vi "Type to String.vi"(7 "application reference (local)":refnum<vi>, 8 "Error In":errorcluster, 11 "Type":variant) -> (0 "Error Out":errorcluster, 3 "String":string)   [LabVIEW 2015, in "Scripting.lvlib"]
uses:
  Scripting.lvlib
  <vilib>/Utility/Data Type/NI_Data Type.lvlib
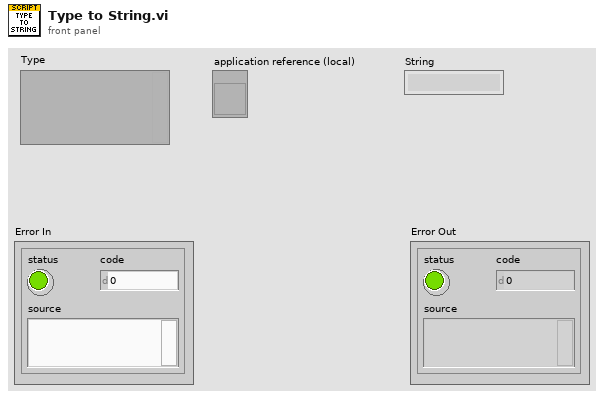
[diagram p1: front panel]
types:
  T1 = typedef "NI_Data Type.lvlib/Data Type.ctl" = enum8{"Invalid Type", "Void", "I8", "I16", "I32", "I64", "U8", "U16", "U32", "U64", "Single Float", "Double Float", "Extended Float", "Single Complex", "Double Complex", "Extended Complex", "Enum U8", "Enum U16", "Enum U32", "Enum U64", "Single Float With Unit", "Double Float With Unit", "Extended Float With Unit", "Single Complex with Unit", "Double Complex with Unit", "Extended Complex with Unit", "Boolean", "String", "Path", "Picture", "Tag", "Array", "Cluster", "Variant", "LV Variant", "Waveform", "Timestamp", "Digital Waveform", "Digital Data", "ExpressData", "Refnum", "External Data", "VI", "Poly VI", "LabVIEW Class Instance", "Fixed Point"}
  T2 = typedef "NI_Data Type.lvlib/Type Definition Info.ctl" = cluster{"Name":string, "Timestamp":u32}
  T3 = cluster{"Unit Type":enum8{"Radians", "Steradians", "Seconds", "Meters", "Kilograms", "Amperes", "Kelvins", "Moles", "Candelas", "InvalidUnit"}, "Exponent":i8}[]
  T4 = cluster{"Type":enum8{"Variable", "Fixed", "Bounded"}, "Size":u32}[]
  T5 = typedef "NI_Data Type.lvlib/Unit Info.ctl" = cluster{"Unit Type":T6, "Exponent":i16}
  T6 = typedef "NI_Data Type.lvlib/Unit Type.ctl" = enum16{"Radians", "Steradians", "Seconds", "Meters", "Kilograms", "Amperes", "Kelvins", "Moles", "Candelas", "InvalidUnit"}
  T7 = typedef "NI_Data Type.lvlib/Memory Info.ctl" = cluster{"Type":T8, "Size":u32}
  T8 = typedef "NI_Data Type.lvlib/Memory Type.ctl" = enum16{"Variable", "Fixed", "Bounded"}
  T9 = cluster{"string":string, string, "string":string}
  T10 = typedef "LVFixedPointRepRangeTypeDef.ctl" = cluster{"Range Min":dbl, "Range Max":dbl, "Delta":dbl}
  T11 = typedef "LVFixedPointRepBitsTypeDef.ctl" = cluster{"Signed":bool, "Word Length":u32, "Integer Word Length":i32}
  T12 = cluster{"FXP Representation":T11, "FXP Range":T10, "Include Overflow Status?":bool}
  T13 = typedef "NI_Data Type.lvlib/Tag Type.ctl" = enum16{"kNoTagType", "\tkDSCTagType", "\tkOldDAQTagType", "\tkIVITagType", "\tkVISATagType", "\tkGenClassTagType", "\tkUnusedTagType1", "\tkFPTagType", "\tkMotionTagType", "\tkDAQmxTaskTagType", "\tkDAQmxChannelTagType", "\tkDAQmxScaleTagType", "\tkDAQmxDeviceTagType", "\tkDAQmxTerminalTagType", "\tkDAQmxPhysChanTagType", "\tkDAQmxTriggerTagType", "\tkDAQmxSwitchTagType", "\tkDAQmxSignalTagType", "\tkUnusedTagType2", "\tkCANTaskTagType", "\tkCANInterfaceTagType", "\tkCANChannelTagType", "\tkNumTagTypes"}
  T14 = typedef "NI_Data Type.lvlib/Refnum Type.ctl" = enum16{"NotARefnum", "UnknownRefnum", "Generic", "Datalog", "ByteStream", "Device", "Occurence", "TCPNetConnection", "Auto", "Menu", "Imaq", "Hardware", "DataSocket", "Visa", "IVI", "UDPNetConnection", "Notifier", "Queue", "Irda", "EventReg", "DotNet", "UserEvent", "Callback", "UNUSED_EMPTY_POSITION", "BlueToothNetConnection", "LVObjApp", "LVObjVI", "LVObjUnknown", "GenericClass", "UserDefinedRefnumTag", "DataValue", "RT FIFO", "TDMS File"}
  T15 = typedef "NI_Data Type.lvlib/VI Info.ctl" = cluster{"Connector Pane Pattern":i16, "Connector Pane Rotation":i16, "Flags":u32[], "Modification Date":timestamp, "Asynchronous":bool, "Non-Function":bool, "Subroutine":bool, "SubSystem":bool}
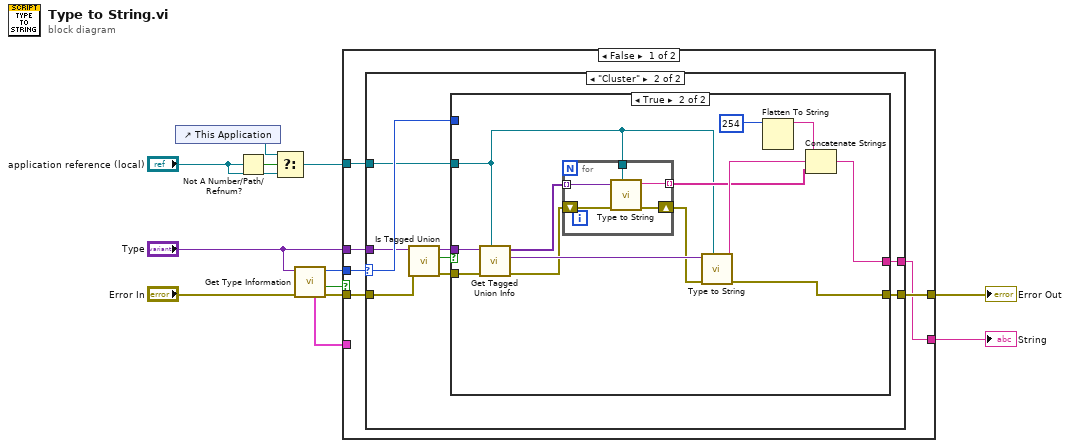
[diagram p0: block diagram]
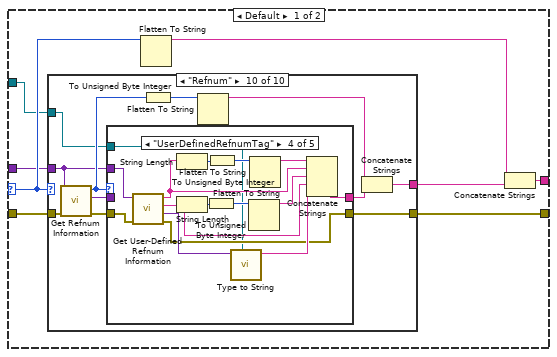
[diagram p2: hidden frame]
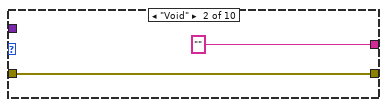
[diagram p4: hidden frame]
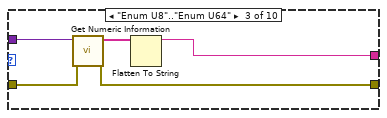
[diagram p5: hidden frame]
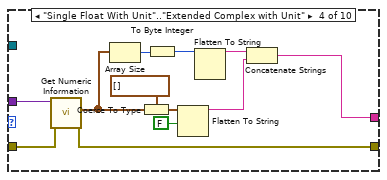
[diagram p6: hidden frame]
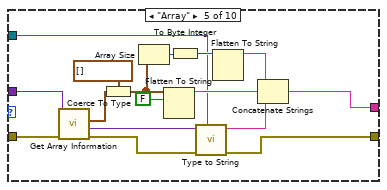
[diagram p7: hidden frame]
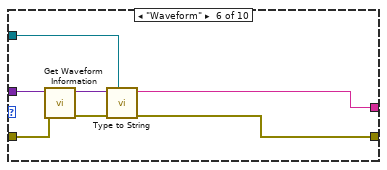
[diagram p8: hidden frame]
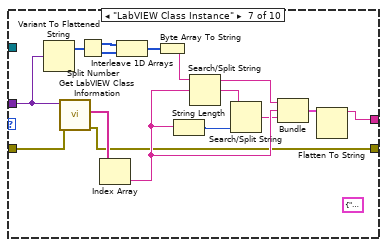
[diagram p9: hidden frame]
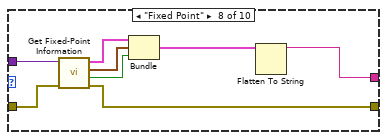
[diagram p10: hidden frame]
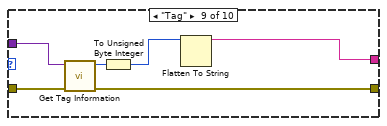
[diagram p11: hidden frame]
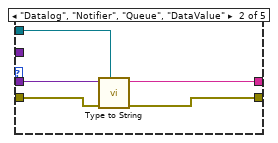
[diagram p13: hidden frame]
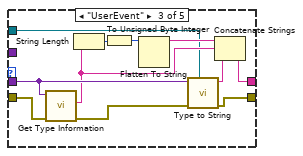
[diagram p14: hidden frame]
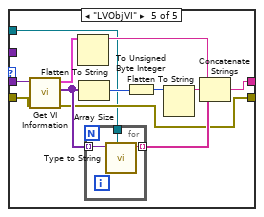
[diagram p15: hidden frame]
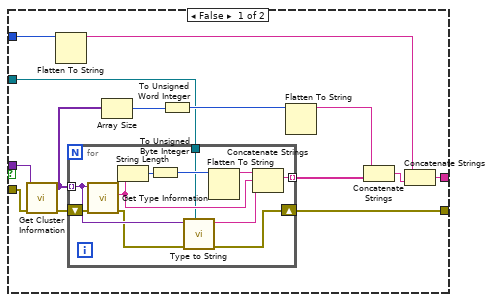
[diagram p16: hidden frame]
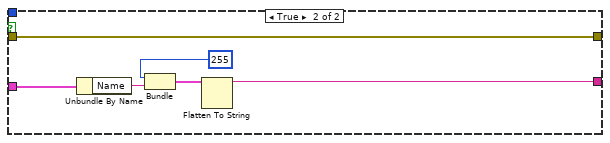
[diagram p17: hidden frame]
diagram:
  n1 = control-ref of="This Application"() -> (w3:refnum<vi>)
  n2 = Not A Number/Path/Refnum?(number/path/refnum="application reference (local)") -> (NaN/Path/Refnum?=w4:bool)
  n3 = Select(t=w3, s=w4, f="application reference (local)") -> (s? t:f=w1:refnum<vi>)
  n4 = call <vilib>:"Get Type Information.vi"("error in (no error)"="Error In", "Variant"="Type") -> ("error out"=w7:errorcluster, "Type Definition"=w11:bool, "Type"=w8:T1, "Type Definition Info"=w10:T2)  [unwired: 5 in, 1 out]
  n5 = case shown="False" w11 {
    tunnel: w10 -> [_ w215]
    tunnel: "Type" -> [w17 _]
    tunnel: w8 -> [w18 _]
    tunnel: w7 -> [w15 w210]
    tunnel: [w14 w211] -> w5
    tunnel: [w16 w210] -> w6
    tunnel: w1 -> [w13 _]
    frame False {
      n6 = case shown="\"Cluster\"" w18 {
        selector: w18 -> [w24 w164]
        tunnel: w17 -> [w20 w161]
        tunnel: [w26 w166] -> w16
        tunnel: w15 -> [w25 w165]
        tunnel: [w21 w163] -> w14
        tunnel: w13 -> [w19 w158]
        frame Default {
          n7 = case shown="\"Refnum\"" w24 {
            tunnel: [w27 w29 w30 w44 w58 w64 w70 w86 w98 w102] -> w26
            tunnel: w25 -> [w27 w29 w31 w45 w62 w69 w85 w92 w99 w110]
            tunnel: [_ "" w34 w35 w55 w65 w83 w87 w94 w104] -> w23
            tunnel: w20 -> [_ _ w33 w46 w61 w68 w82 w93 w97 w101]
            tunnel: w19 -> [_ _ _ _ w47 w63 _ _ _ w100]
            frame Default {
            }
            frame "Void" {
            }
            frame "Enum U8".."Enum U64" {
              n8 = call <vilib>:"Get Numeric Information.vi"("error in (no error)"=w31, "Variant"=w33) -> ("error out"=w30:errorcluster, "Enum Names"=w32:string[])  [unwired: 6 in, 2 out]
              n9 = Flatten To String(anything=w32) -> (data string=w34:string)  [unwired: 3 in, 2 out]
            }
            frame "Single Float With Unit".."Extended Complex with Unit" {
              n10 = call <vilib>:"Get Numeric Information.vi"("error in (no error)"=w45, "Variant"=w46) -> ("error out"=w44:errorcluster, "Units"=w40:T5[])  [unwired: 6 in, 2 out]
              n11 = Array Size(array=w40) -> (size(s)=w39:i32)
              n12 = Coerce To Type(0:w40, 1:T3 [] ("type")) -> (2:w42:T3)
              n13 = To Byte Integer(number=w39) -> (8bit integer=w38:i8)
              n14 = Flatten To String(anything=w42, prepend array or string size? (T)=FALSE) -> (data string=w36:string)  [unwired: 2 in, 2 out]
              n15 = Flatten To String(anything=w38) -> (data string=w37:string)  [unwired: 3 in, 2 out]
              n16 = Concatenate Strings(w37, w36) -> (w35:string)
            }
            frame "Array" {
              n17 = call <vilib>:"Get Array Information.vi"("error in (no error)"=w62, "Variant"=w61) -> ("error out"=w59:errorcluster, "Array Element Data Type"=w60:variant, "Array Lengths"=w54:T7[])  [unwired: 6 in, 1 out]
              n18 = Coerce To Type(0:w54, 1:T4 [] ("Array Lengths")) -> (2:w51:T4)
              n19 = Array Size(array=w51) -> (size(s)=w50:i32)
              n20 = Flatten To String(anything=w51, prepend array or string size? (T)=FALSE) -> (data string=w57:string)  [unwired: 2 in, 2 out]
              n21 = To Byte Integer(number=w50) -> (8bit integer=w49:i8)
              n22 = call "Type to String.vi"("application reference (local)"=w47, "Error In"=w59, "Type"=w60) -> ("Error Out"=w58:errorcluster, "String"=w56:string)  [unwired: 7 in]
              n23 = Flatten To String(anything=w49) -> (data string=w48:string)  [unwired: 3 in, 2 out]
              n24 = Concatenate Strings(w48, w57, w56) -> (w55:string)
            }
            frame "Waveform" {
              n25 = call <vilib>:"Get Waveform Information.vi"("error in (no error)"=w69, "Variant"=w68) -> ("error out"=w66:errorcluster, "Y Array Type"=w67:variant)  [unwired: 8 in]
              n26 = call "Type to String.vi"("application reference (local)"=w63, "Error In"=w66, "Type"=w67) -> ("Error Out"=w64:errorcluster, "String"=w65:string)  [unwired: 7 in]
            }
            frame "LabVIEW Class Instance" {
              (unwired) T9 {"string"="", "", "string"=""} ("output cluster")
              n27 = Variant To Flattened String(Variant=w82) -> (1:w81:i16[])  [unwired: 1 out]
              n28 = call <vilib>:"Get LabVIEW Class Information.vi"("error in (no error)"=w85, "Variant"=w82) -> ("error out"=w70:errorcluster, "Qualified LabVIEW Class Name"=w84:string[])  [unwired: 7 in, 1 out]
              n29 = Split Number(x=w81) -> (hi(x)=w80:u8[], lo(x)=w79:u8[])
              n30 = Index Array(array=w84) -> (element=w73:string)  [unwired: 1 in]
              n31 = Interleave 1D Arrays(w80, w79) -> (w78:u8[])
              n32 = Byte Array To String(unsigned byte array=w78) -> (string=w77:string)
              n33 = String Length(string=w73) -> (length=w75:i32)
              n34 = Search/Split String(string=w77, search string/char (-)=w73) -> (substring before match=w74:string, match + rest of string=w76:string)  [unwired: 1 in, 1 out]
              n35 = Search/Split String(string=w76, offset (0)=w75) -> (match + rest of string=w72:string)  [unwired: 1 in, 2 out]
              n36 = Bundle("string"=w74, w73, "string"=w72) -> (w71:T9)  [unwired: 1 in]
              n37 = Flatten To String(anything=w71) -> (data string=w83:string)  [unwired: 3 in, 2 out]
            }
            frame "Fixed Point" {
              n38 = call <vilib>:"Get Fixed-Point Information.vi"("error in (no error)"=w92, "Variant"=w93) -> ("error out"=w86:errorcluster, "Include Overflow Status?"=w89:bool, "FXP Range"=w90:T10, "FXP Representation"=w91:T11)  [unwired: 6 in]
              n39 = Bundle("FXP Representation"=w91, "FXP Range"=w90, "Include Overflow Status?"=w89) -> (w88:T12)  [unwired: 1 in]
              n40 = Flatten To String(anything=w88) -> (data string=w87:string)  [unwired: 3 in, 2 out]
            }
            frame "Tag" {
              n41 = call <vilib>:"Get Tag Information.vi"("error in (no error)"=w99, "Variant"=w97) -> ("error out"=w98:errorcluster, "Tag Type"=w96:T13)  [unwired: 8 in]
              n42 = To Unsigned Byte Integer(number=w96) -> (unsigned 8bit integer=w95:u8)
              n43 = Flatten To String(anything=w95) -> (data string=w94:string)  [unwired: 3 in, 2 out]
            }
            frame "Refnum" {
              n44 = call <vilib>:"Get Refnum Information.vi"("error in (no error)"=w110, "Variant"=w101) -> ("error out"=w107:errorcluster, "Strict Type"=w106:variant, "Reference Type"=w109:T14)  [unwired: 6 in, 1 out]
              n45 = case shown="\"UserDefinedRefnumTag\"" w109 {
                tunnel: w107 -> [w111 w115 w127 w142 w147]
                tunnel: w106 -> [_ w116 w124 _ w146]
                tunnel: [_ w114 w119 w131 w145] -> w103
                tunnel: [w111 w113 w126 w130 w144] -> w102
                tunnel: w101 -> [_ _ _ w129 _]
                tunnel: w100 -> [_ w112 w117 w128 w143]
                frame Default {
                }
                frame "Datalog", "Notifier", "Queue", "DataValue" {
                  n46 = call "Type to String.vi"("application reference (local)"=w112, "Error In"=w115, "Type"=w116) -> ("Error Out"=w113:errorcluster, "String"=w114:string)  [unwired: 7 in]
                }
                frame "UserEvent" {
                  n47 = call <vilib>:"Get Type Information.vi"("error in (no error)"=w127, "Variant"=w124) -> ("error out"=w125:errorcluster, "Name"=w121:string)  [unwired: 5 in, 3 out]
                  n48 = String Length(string=w121) -> (length=w123:i32)
                  n49 = To Unsigned Byte Integer(number=w123) -> (unsigned 8bit integer=w118:u8)
                  n50 = Flatten To String(anything=w118) -> (data string=w122:string)  [unwired: 3 in, 2 out]
                  n51 = call "Type to String.vi"("application reference (local)"=w117, "Error In"=w125, "Type"=w124) -> ("Error Out"=w126:errorcluster, "String"=w120:string)  [unwired: 7 in]
                  n52 = Concatenate Strings(w122, w121, w120) -> (w119:string)
                }
                frame "UserDefinedRefnumTag" {
                  n53 = call <vilib>:"Get User-Defined Refnum Information.vi"("error in (no error)"=w142, "Variant"=w129) -> ("error out"=w130:errorcluster, "User Data"=w141:variant, "Type Name"=w133:string, "Class Name"=w135:string)  [unwired: 6 in]
                  n54 = String Length(string=w135) -> (length=w138:i32)
                  n55 = String Length(string=w133) -> (length=w137:i32)
                  n56 = To Unsigned Byte Integer(number=w137) -> (unsigned 8bit integer=w139:u8)
                  n57 = To Unsigned Byte Integer(number=w138) -> (unsigned 8bit integer=w140:u8)
                  n58 = call "Type to String.vi"("application reference (local)"=w128, "Type"=w141) -> ("String"=w132:string)  [unwired: 8 in, 1 out]
                  n59 = Flatten To String(anything=w139) -> (data string=w134:string)  [unwired: 3 in, 2 out]
                  n60 = Flatten To String(anything=w140) -> (data string=w136:string)  [unwired: 3 in, 2 out]
                  n61 = Concatenate Strings(w136, w135, w134, w133, w132) -> (w131:string)
                }
                frame "LVObjVI" {
                  n62 = call <vilib>:"Get VI Information.vi"("error in (no error)"=w147, "Variant"=w146) -> ("error out"=w144:errorcluster, "VI Terminal Types"=w149:variant[], "VI Info"=w148:T15)  [unwired: 6 in, 1 out]
                  n63 = Flatten To String(anything=w148) -> (data string=w152:string)  [unwired: 3 in, 2 out]
                  n64 = Array Size(array=w149) -> (size(s)=w150:i32)
                  n65 = for {
                    tunnel: w149 -> [w157] mode=indexing
                    tunnel: [w156] -> w154 mode=indexing
                    tunnel: w143 -> [w155]
                    n66 = call "Type to String.vi"("application reference (local)"=w155, "Type"=w157) -> ("String"=w156:string)  [unwired: 8 in, 1 out]
                  }
                  n67 = To Unsigned Byte Integer(number=w150) -> (unsigned 8bit integer=w151:u8)
                  n68 = Flatten To String(anything=w151) -> (data string=w153:string)  [unwired: 3 in, 2 out]
                  n69 = Concatenate Strings(w152, w153, w154) -> (w145:string)
                }
              }
              n70 = To Unsigned Byte Integer(number=w109) -> (unsigned 8bit integer=w108:u8)
              n71 = Flatten To String(anything=w108) -> (data string=w105:string)  [unwired: 3 in, 2 out]
              n72 = Concatenate Strings(w105, w103) -> (w104:string)
            }
          }
          n73 = Flatten To String(anything=w24) -> (data string=w22:string)  [unwired: 3 in, 2 out]
          n74 = Concatenate Strings(w22, w23) -> (w21:string)
        }
        frame "Cluster" {
          n75 = call "Is Tagged Union.vi"("Error In"=w165, "Type in"=w161) -> ("Error Out"=w162:errorcluster, "Tagged Union?"=w159:bool, "Type out"=w160:variant)  [unwired: 7 in]
          n76 = case shown="True" w159 {
            tunnel: [w180 w193] -> w166
            tunnel: w162 -> [w179 w203]
            tunnel: w164 -> [w178 _]
            tunnel: [w175 w198] -> w163
            tunnel: w160 -> [w174 w204]
            tunnel: w158 -> [w167 w192]
            frame False {
              n77 = call <vilib>:"Get Cluster Information.vi"("error in (no error)"=w179, "Variant"=w174) -> ("error out"=w173:errorcluster, "Cluster Elements"=w171:variant[])  [unwired: 8 in]
              n78 = Flatten To String(anything=w178) -> (data string=w176:string)  [unwired: 3 in, 2 out]
              n79 = for {
                tunnel: w171 -> [w189] mode=indexing
                tunnel: [w184] -> w168 mode=indexing
                shift-right: [w191] -> w180
                shift-left: w173 -> [w190]
                tunnel: w167 -> [w181]
                n80 = call <vilib>:"Get Type Information.vi"("error in (no error)"=w190, "Variant"=w189) -> ("error out"=w188:errorcluster, "Name"=w182:string)  [unwired: 5 in, 3 out]
                n81 = String Length(string=w182) -> (length=w187:i32)
                n82 = To Unsigned Byte Integer(number=w187) -> (unsigned 8bit integer=w186:u8)
                n83 = call "Type to String.vi"("application reference (local)"=w181, "Error In"=w188, "Type"=w189) -> ("Error Out"=w191:errorcluster, "String"=w183:string)  [unwired: 7 in]
                n84 = Flatten To String(anything=w186) -> (data string=w185:string)  [unwired: 3 in, 2 out]
                n85 = Concatenate Strings(w185, w182, w183) -> (w184:string)
              }
              n86 = Array Size(array=w171) -> (size(s)=w170:i32)
              n87 = To Unsigned Word Integer(number=w170) -> (unsigned 16bit integer=w172:u16)
              n88 = Flatten To String(anything=w172) -> (data string=w169:string)  [unwired: 3 in, 2 out]
              n89 = Concatenate Strings(w169, w168) -> (w177:string)
              n90 = Concatenate Strings(w176, w177) -> (w175:string)
            }
            frame True {
              n91 = call "Get Tagged Union Info.vi"("application reference (local)"=w192, "error in (no error)"=w203, "Type in"=w204) -> ("error out"=w194:errorcluster, "Enum Type"=w202:variant, "Element Types"=w197:variant[])  [unwired: 6 in]
              n92 = for {
                tunnel: w197 -> [w209] mode=indexing
                tunnel: [w208] -> w196 mode=indexing
                shift-right: [w206] -> w195
                shift-left: w194 -> [w207]
                tunnel: w192 -> [w205]
                n93 = call "Type to String.vi"("application reference (local)"=w205, "Error In"=w207, "Type"=w209) -> ("Error Out"=w206:errorcluster, "String"=w208:string)  [unwired: 7 in]
              }
              n94 = call "Type to String.vi"("application reference (local)"=w192, "Error In"=w195, "Type"=w202) -> ("Error Out"=w193:errorcluster, "String"=w199:string)  [unwired: 7 in]
              n95 = Flatten To String(anything=u8 254) -> (data string=w200:string)  [unwired: 3 in, 2 out]
              n96 = Concatenate Strings(w200, w199, w196) -> (w198:string)
            }
          }
        }
      }
    }
    frame True {
      n97 = Unbundle By Name(w215) -> ("Name"=w214:string)
      n98 = Bundle(u8 255, "Name"=w214) -> (w212:cluster{u8, "Name":string})  [unwired: 1 in]
      n99 = Flatten To String(anything=w212) -> (data string=w211:string)  [unwired: 3 in, 2 out]
    }
  }
  "Error Out" <- w6
  "String" <- w5
